vi "Demo.vi"() -> ()   [LabVIEW 2014]
uses:
  1/ExampleClass.lvclass
  2/ExampleClass2.lvclass
  2/ExampleClass2.lvclass/ExampleClass2.ctl
  1/ExampleClass.lvclass/ExampleClass.ctl
  Singleton/Singleton.lvclass
panel:
  in  "Numeric":dbl=134.0
  in  "Numeric 1":dbl=12345.0
  in  "stop":bool
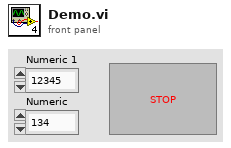
[diagram p1: front panel]
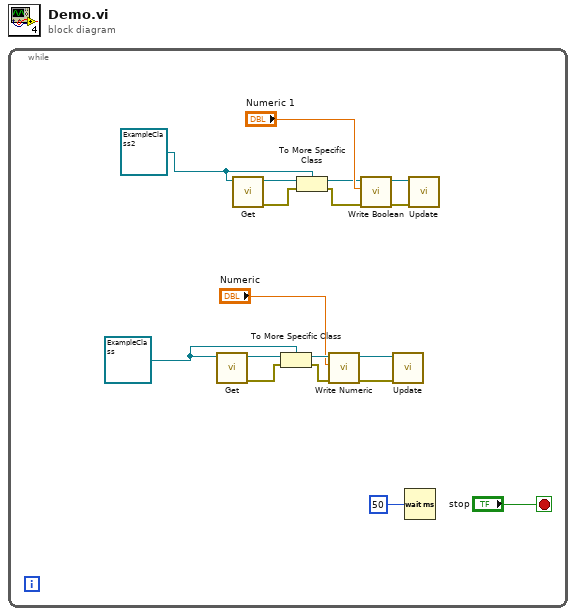
[diagram p0: block diagram]
diagram:
  n1 = while {
    stop <- "stop" stop-if-true
    w15 = refnum<class "ExampleClass2.lvclass"> refnum ("ExampleClass2")
    w8 = refnum<class "ExampleClass.lvclass"> refnum ("ExampleClass")
    n2 = call "Get.vi"("Template"=w8) -> ("error out"=w5:errorcluster, "object"=w2:refnum<class "Singleton.lvclass">)  [unwired: 9 in]
    n3 = call "Get.vi"("Template"=w15) -> ("error out"=w11:errorcluster, "object"=w14:refnum<class "Singleton.lvclass">)  [unwired: 9 in]
    n4 = To More Specific Class(target class=w8, reference=w2, error in=w5) -> (specific class reference=w3:refnum<class "ExampleClass.lvclass">, error out=w4:errorcluster)
    n5 = To More Specific Class(target class=w15, reference=w14, error in=w11) -> (specific class reference=w13:refnum<class "ExampleClass2.lvclass">, error out=w12:errorcluster)
    n6 = call "Write Numeric.vi"("error in (no error)"=w4, "Numeric"="Numeric", "ExampleClass in"=w3) -> ("error out"=w6:errorcluster, "ExampleClass out"=w7:refnum<class "ExampleClass.lvclass">)  [unwired: 7 in]
    n7 = call "Write Boolean.vi"("error in (no error)"=w12, "Numeric"="Numeric 1", "ExampleClass2 in"=w13) -> ("error out"=w10:errorcluster, "ExampleClass2 out"=w9:refnum<class "ExampleClass2.lvclass">)  [unwired: 7 in]
    n8 = call "Update.vi"("error in (no error)"=w6, "Object"=w7) -> ()  [unwired: 8 in, 2 out]
    n9 = Wait (ms)(milliseconds to wait=u32 50) -> ()  [unwired: 1 out]
    n10 = call "Update.vi"("error in (no error)"=w10, "Object"=w9) -> ()  [unwired: 8 in, 2 out]
  }
